vi "ABB Test HV.vi"() -> ()   [LabVIEW 2017]
uses:
  ABB global.vi
panel:
  in  "Rotor Insulation Resistance":T1
  in  "Stator Insulation Resistance":T1
  out "Motor Type":string
  out "Serial number":string
  out "W.O number":string
  out "Timedate":string
  in  "Exit":bool
  # "High Voltage Test"
  # "with"
  # "at"
  # "with"
  # "at"
  # "with"
  # "at"
  # "at"
  # "with"
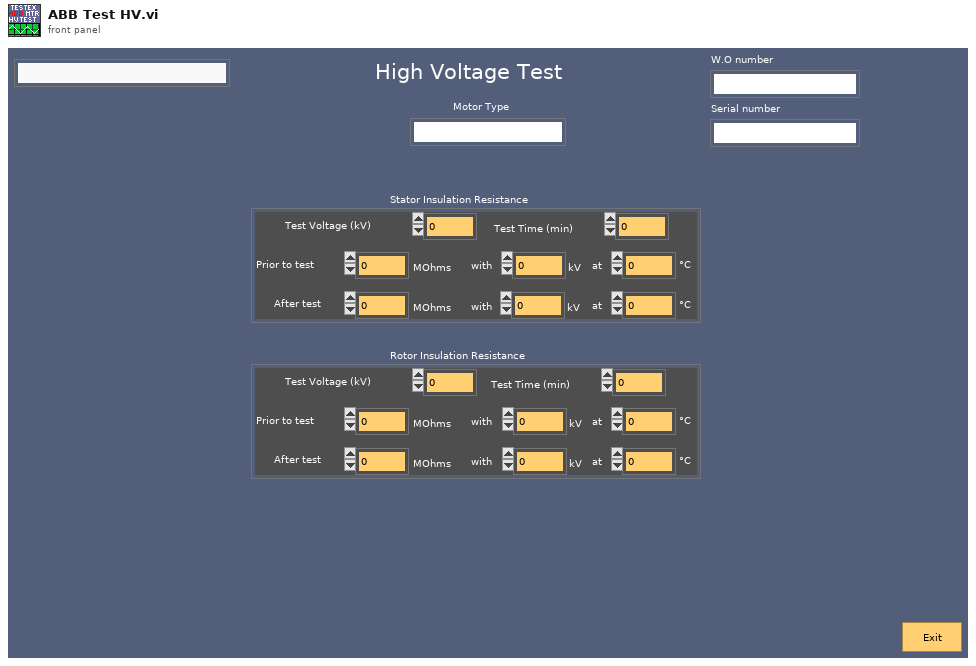
[diagram p1: front panel]
types:
  T1 = cluster{"Prior to test":dbl, "Prior v":dbl, "Prior temp":dbl, "After test":dbl, "after v":dbl, "After temp":dbl, "Test Voltage (kV)":dbl, "Test Time (min)":dbl}
  T2 = cluster{"Simulate Norma":bool, "Norma 5000 Address":u8, "WebDaq IP Address":string, "Simulate cDAQ":bool}
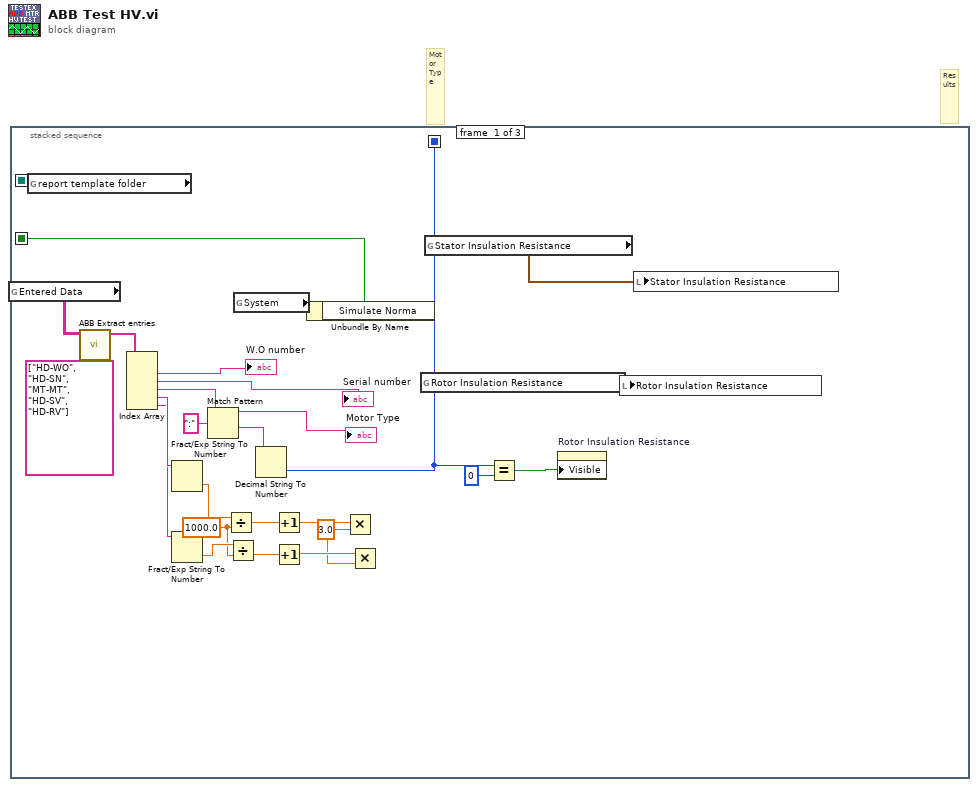
[diagram p0: block diagram]
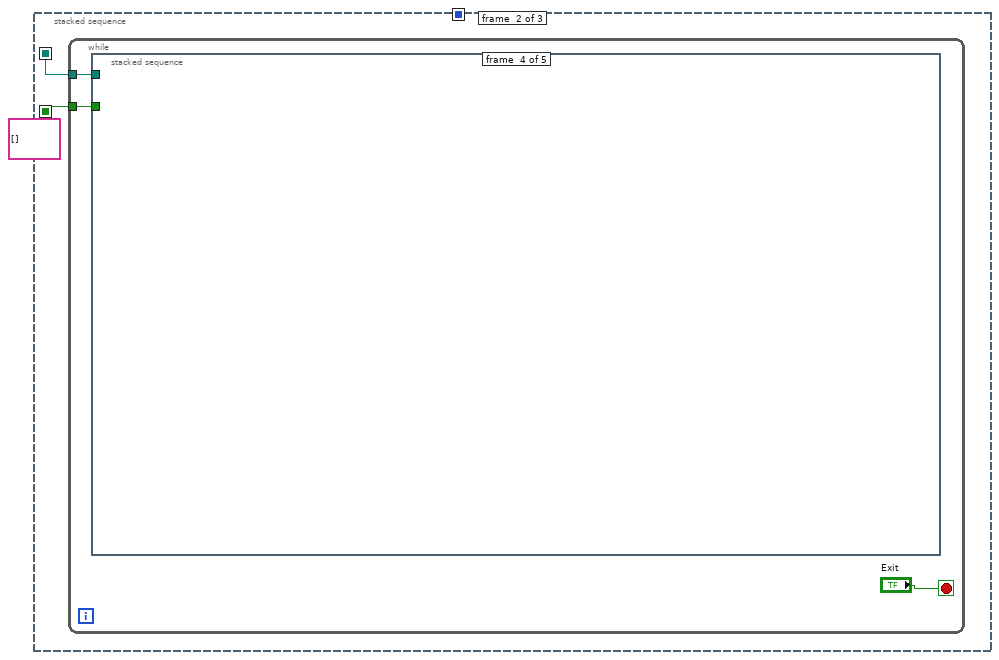
[diagram p2: hidden frame]
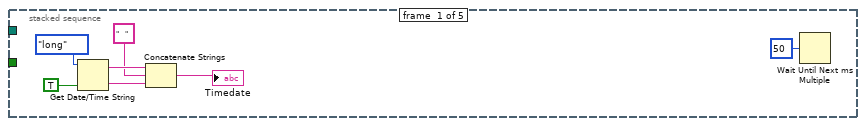
[diagram p3: hidden frame]
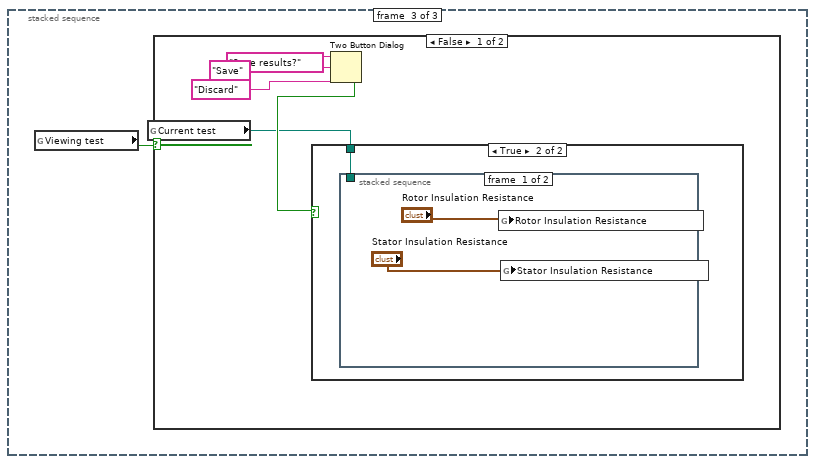
[diagram p7: hidden frame]
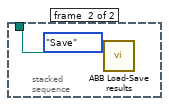
[diagram p9: hidden frame]
diagram:
  # "Motor Type"
  # "Results"
  n1 = stacked-sequence {
    seq-local: [w26 _ _] -> [_ w29 _]
    seq-local: [w21 _ _] -> [_ w28 _]
    seq-local: [w15 _ _] -> [_ _ _]
    frame #0 {
      w2 = 3.0 ("y")
      w7 = 1000.0 ("y")
      n2 = global read "ABB global.vi" "Entered Data"() -> (w20:string[][])
      n3 = global read "ABB global.vi" "report template folder"() -> (w21:path)
      n4 = call "ABB Extract entries.vi"("Entry IDs"=string[] ["HD-WO", "HD-SN", "MT-MT", "HD-SV", "HD-RV"], "Entry table in"=w20) -> ("Selected Entries"=w25:string[])  [unwired: 9 in]
      n5 = Index Array(array=w25) -> (element #1=→"W.O number":string, element #2=→"Serial number":string, element #3=w19:string, element #4=w11:string, element #5=w9:string)  [unwired: 5 in]
      n6 = Fract/Exp String To Number(string=w11) -> (number=w10:dbl)  [unwired: 3 in, 1 out]
      n7 = Fract/Exp String To Number(string=w9) -> (number=w8:dbl)  [unwired: 3 in, 1 out]
      n8 = Match Pattern(string=w19, regular expression=":") -> (before substring=→"Motor Type":string, after substring=w16:string)  [unwired: 1 in, 2 out]
      n9 = Divide(x=w10, y=w7) -> (x/y=w6:dbl)
      n10 = Divide(x=w8, y=w7) -> (x/y=w5:dbl)
      n11 = global read "ABB global.vi" "System"() -> (w27:T2)
      n12 = Decimal String To Number(string=w16) -> (number=w15:i32)  [unwired: 2 in, 1 out]
      n13 = Increment(x=w6) -> (x+1=w4:dbl)
      n14 = Increment(x=w5) -> (x+1=w3:dbl)
      n15 = Unbundle By Name(w27) -> ("Simulate Norma"=w26:bool)
      n16 = Multiply(x=w4, y=w2) -> ()  [unwired: 1 out]
      n17 = Multiply(x=w3, y=w2) -> ()  [unwired: 1 out]
      n18 = global read "ABB global.vi" "Rotor Insulation Resistance"() -> (w12:T1)
      n19 = global read "ABB global.vi" "Stator Insulation Resistance"() -> (w1:T1)
      n20 = Equal?(x=w15, y=0) -> (x = y?=w13:bool)
      n21 = property on="Rotor Insulation Resistance" class="Clust (strict)"("Visible"=w13) -> ()  [unwired: 2 in, 2 out]
      n22 = local write "Rotor Insulation Resistance"(w12) -> ()
      n23 = local write "Stator Insulation Resistance"(w1) -> ()
    }
    frame #1 {
      (unwired) string[][] [] ("Cooling Curve Data")
      n24 = while {
        tunnel: w29 -> [w31]
        tunnel: w28 -> [w30]
        stop <- "Exit" stop-if-true
        n25 = stacked-sequence {
          tunnel: w31 -> [_ _ _ _ _]
          tunnel: w30 -> [_ _ _ _ _]
          frame #0 {
            n26 = Get Date/Time String(date format (0)=enum16{"short", "long", "abbreviated"}."long", want seconds? (F)=TRUE) -> (date string=w37:string, time string=w36:string)  [unwired: 1 in]
            n27 = Concatenate Strings(w37, "   ", w36) -> (→"Timedate":string)
            n28 = Wait Until Next ms Multiple(millisecond multiple=u32 50) -> ()  [unwired: 1 out]
          }
          frame #1 {
          }
          frame #2 {
          }
          frame #3 {
          }
          frame #4 {
          }
        }
      }
    }
    frame #2 {
      n29 = global read "ABB global.vi" "Viewing test"() -> (w40:bool)
      n30 = case shown="False" w40 {
        frame False {
          n31 = global read "ABB global.vi" "Current test"() -> (w43:path)
          n32 = Two Button Dialog(message="Save results?", 1:"Discard" ("F button name (\"Cancel\")"), 2:"Save" ("T button name (\"OK\")")) -> (T button?=w44:bool)
          n33 = case shown="True" w44 {
            tunnel: w43 -> [_ w46]
            frame False {
            }
            frame True {
              n34 = stacked-sequence {
                tunnel: w46 -> [_ w49]
                frame #0 {
                  n35 = global write "ABB global.vi" "Rotor Insulation Resistance"("Rotor Insulation Resistance") -> ()
                  n36 = global write "ABB global.vi" "Stator Insulation Resistance"("Stator Insulation Resistance") -> ()
                }
                frame #1 {
                  n37 = call "ABB Load-Save results.vi"("Path"=w49, "Mode"=enum16{"LOAD", "Save"}."Save") -> ()  [unwired: 10 in]
                }
              }
            }
          }
        }
        frame True {
        }
      }
    }
  }
